vi "acquire_FXP_18-5_FIFO_1.vi"(6 "numChannels":i16, 7 "Iters":i32, 8 "error in":errorcluster, 11 "FPGA Interface":T1) -> (0 "error out":errorcluster, 1 "Elements Remaining":u32, 2 "2D Data Out":dbl[][](array[numeric]), 3 "acquisition done":bool, 5 "u iter":i32)   [LabVIEW 2017]
uses:
  fpga_interface_types/FPGA_to_HOST_1_FXP_18-5_FIFO_interface.ctl
  <vilib>/Utility/error.llb/Error Cluster From Error Code.vi
  <vilib>/rvi/errors/niLvFpgaAdjustHostInterfaceError.vi
  <vilib>/rvi/interface/nirviMethod/nirviMethod.xnode
  <vilib>/FPGAPlugInAG/Dynamic/niLvFpga_ReadFifo_Dynamic.vi
  <vilib>/rvi/errors/niLvFpgaMergeErrorWithErrorCode.vi
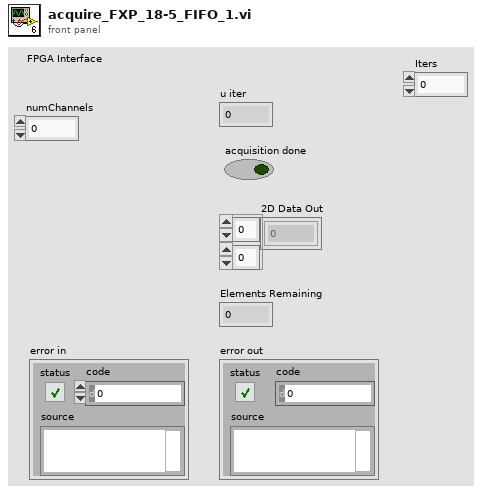
[diagram p1: front panel]
types:
  T1 = typedef "FPGA_to_HOST_1_FXP_18-5_FIFO_interface.ctl" = refnum<k20>
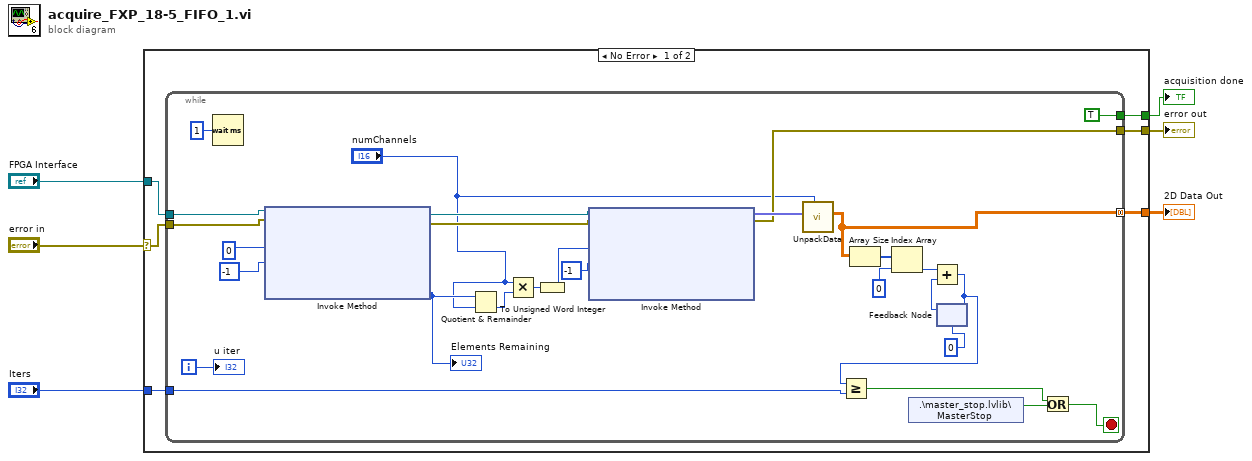
[diagram p0: block diagram]
diagram:
  n1 = case shown="No Error" "error in" {
    selector: "error in" -> [w7 w41]
    tunnel: [w12 _] -> w6
    tunnel: [w11 w41] -> w5
    tunnel: [w10 _] -> w4
    tunnel: "Iters" -> [w9 _]
    tunnel: "FPGA Interface" -> [w8 _]
    frame No Error {
      n2 = while {
        tunnel: [w34] -> w10 mode=concatenating
        tunnel: w8 -> [w28]
        tunnel: w7 -> [w27]
        tunnel: [w25] -> w11
        tunnel: [TRUE] -> w12
        tunnel: w9 -> [w15]
        i -> [w36]
        stop <- w20 stop-if-true
        n3 = Wait (ms)(milliseconds to wait=u32 1) -> ()  [unwired: 1 out]
        n4 = xnode "Invoke Method"("FPGA VI Reference In"=w28, "error in"=w27, "Number of Elements"=0 ("Timeout (ms)"), "Timeout (ms)"=-1) -> ("FPGA VI Reference Out"=w21:T1, "error out"=w24:errorcluster, "Elements Remaining"=w31:u32)  [unwired: 1 out]
        "Elements Remaining" <- w31
        n5 = Quotient & Remainder(x=w31, y="numChannels") -> (floor(x/y)=w38:u32)  [unwired: 1 out]
        n6 = Multiply(x="numChannels", y=w38) -> (x*y=w39:u32)
        n7 = To Unsigned Word Integer(number=w39) -> (unsigned 16bit integer=w23:u16)
        n8 = xnode "Invoke Method"("FPGA VI Reference In"=w21, "error in"=w24, "Number of Elements"=w23, "Timeout (ms)"=-1) -> ("error out"=w25:errorcluster, "Data"=w26:fxp<+/-,18,5>[])  [unwired: 2 out]
        n9 = call "UnpackData.vi"("NumChannels"="numChannels", "1D Data In"=w26) -> ("2D Data Out"=w34:dbl[][])  [unwired: 8 in, 1 out]
        n10 = Array Size(array=w34) -> (size(s)=w32:i32[])
        n11 = Index Array(array=w32, index=0) -> (element=w35:i32)
        n12 = shared-variable ".\\master_stop.lvlib\\MasterStop"() -> (w18:bool)  [unwired: 1 in, 1 out]
        n13 = feedback #1(0) -> (w37:i32)
        n14 = Add(x=w35, y=w37) -> (x+y=w16:i32)
        n15 = Greater Or Equal?(x=w16, y=w15) -> (x >= y?=w19:bool)
        n16 = feedback-in #1(w16) -> ()
        n17 = Or(x=w19, y=w18) -> (x .or. y?=w20:bool)
        "u iter" <- w36
      }
    }
    frame Error {
    }
  }
  "acquisition done" <- w6
  "error out" <- w5
  "2D Data Out" <- w4
